vi "Randomness.vi"(8 "error in (no error)":errorcluster, 10 "nbytes":i32) -> (0 "error out":errorcluster, 2 "random bytes":u8[](array[numeric]) format="%.0x")   [LabVIEW 2014, in "SQLite3LV.lvlib" / "sqlite3.lvclass"]
doc: "void SQLite3LV Connection_randomness(int N, void *P);\n\nSQLite contains a high-quality pseudo-random number generator (PRNG) used to select random ROWIDs when inserting new records into a table that already uses the largest possible ROWID. The PRNG is also used for the build-in random() and randomblob() SQL functions. This interface allows applications to access the same PRNG for other purposes.\n\nA call to this routine stores N bytes of randomness into buffer P. The P parameter can be a NULL pointer.\n\nIf this routine has not been previously called or if the previous call had N less than one or a NULL pointer for P, then the PRNG is seeded using randomness obtained from the xRandomness method of the default sqlite3_vfs object. If the previous call to this routine had an N of 1 or more and a non-NULL P then the pseudo-randomness is generated internally and without recourse to the sqlite3_vfs xRandomness method."
uses:
  sqlite3.lvclass
  sqlite3_64.dll
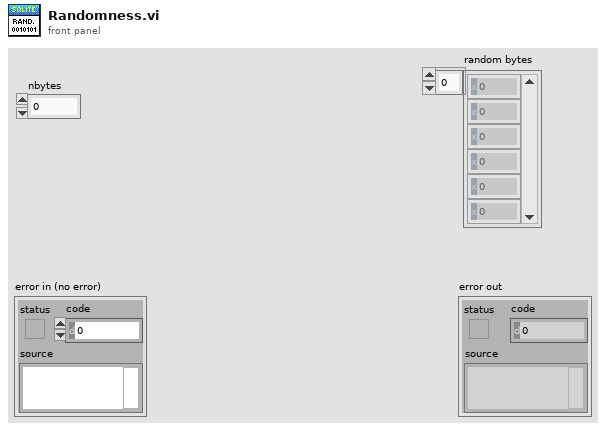
[diagram p1: front panel]
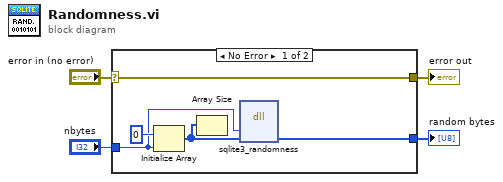
[diagram p0: block diagram]
diagram:
  n1 = case shown="No Error" "error in (no error)" {
    selector: "error in (no error)" -> [w9 w10]
    tunnel: [w9 w10] -> w3
    tunnel: "nbytes" -> [w5 _]
    tunnel: [w8 _] -> w1
    frame No Error {
      n2 = Initialize Array(u8 0, w5) -> (w6:u8[])
      n3 = Array Size(array=w6) -> ()  [unwired: 1 out]
      n4 = dll-call lib="C:/Users/BobUser/Desktop/LVTables/sqlite3**.*" fn="sqlite3_randomness"("nBytes"=w5, "pData"=w6) -> ("pData"=w8:u8[])  [unwired: 5 in, 2 out]
    }
    frame Error {
    }
  }
  "error out" <- w3
  "random bytes" <- w1
